vi "Max Time Acceleration.vi"(1 "Max Acceleration":dbl, 2 "Max Velocity":dbl) -> (0 "Max Time Acceleration":dbl)   [LabVIEW 2015]
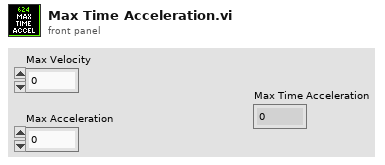
[diagram p1: front panel]
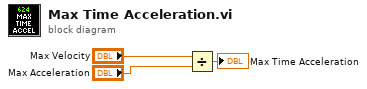
[diagram p0: block diagram]
diagram:
  n1 = Divide(x="Max Velocity", y="Max Acceleration") -> (x/y=→"Max Time Acceleration":dbl)
